vi "加标回收启动 (子VI).vi"(11 "启动参数":T1(ring)=enum."CODCr") -> (0 "error out":T2={"status"=FALSE, "代码"=4, "source"=""} caption="错误输出" {"代码" items=["执行成功"=1, "执行失败，但不知道原因"=2, "命令请求条件错误"=3, "通讯超时"=4, "系统繁忙不能执行"=5, "系统故障"=6, "没有数据"=100]})   [LabVIEW 2016]
uses:
  PLC/PLC.lvlib
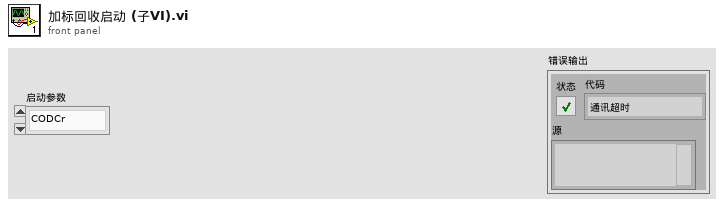
[diagram p1: front panel]
types:
  T1 = enum16{"未选择", "CODMn", "氨氮", "总磷", "总氮", "CODCr"}
  T2 = cluster{"status":bool, "代码":u16, "source":string}
  T3 = enum16{"空闲", "水样测试", "标样核查", "零点核查", "跨度核查", "空白测试", "平行样测试", "质控样", "空白校准", "标样校准", "加标回收"}
  T4 = enum16{"空闲", "水样测试", "标样核查", "零点核查", "跨度核查", "空白测试", "平行样测试", "加标回收", "空白校准", "标样校准", "初始化（清洗）"}
  T5 = cluster{"是否启用仪器":bool, "CODMn":cluster{"启动测量模式":cluster{"测量模式":enum16{"水样测量", "标样核查", "加标回收", "平行样", "校零", "校标"}}, "确定按钮":bool}, "启动模块":cluster{"氨氮":bool, "总磷":bool, "总氮":bool, "COD":bool}, "常规启动":bool, "直接启动":bool}
  T6 = cluster{"R0":i16, "R1":i16, "R2":i16, "R3":i16, "R4":i16, "R5":i16, "R6":i16, "R7":i16, "R8":i16, "R9":i16, "R10":i16, "R11":i16, "R12":i16, "R13":i16, "R14":i16, "R15":i16, "R16":i16, "R17":i16, "R18":i16, "R19":i16, "R20":i16, "R21":i16, "R22":i16, "R23":i16, "R24":i16, "R25":i16, "R26":i16, "R27":i16, "R28":i16, "R29":i16, "R30":i16, "R31":i16, "R32":i16, "R33":i16, "R34":i16, "R35":i16, "R36":i16, "R37":i16, "R38":i16, "R39":i16, "R40":i16, "R41":i16, "R42":i16, "R43":i16, "R44":i16, "R45":i16, "R46":i16, "R47":i16, "R48":i16, "R49":i16, "R50":i16, "R51":i16, "R52":i16, "R53":i16, "R54":i16, "R55":i16, "R56":i16}
  T7 = enum32{"Bad", "Idle", "Run top level", "Running"}
  T8 = cluster{"系统时间":timestamp, "工作状态":enum16{"空闲", "水样测试", "标样核查", "零点核查", "跨度核查", "空白测试", "平行样测试", "加标回收", "空白校准", "标样校准", "初始化（清洗）"}, "测量模式":enum16{"待机", "连续模式", "周期模式", "定点模式", "受控模式", "手动模式"}, "告警代码":u16, "故障代码":u16, "日志代码":u16, "软件版本":u16, "F0":sgl, "F1":sgl, "F2":sgl, "F3":sgl, "T":sgl, "H":sgl, "id":u16, "flowid":u16, "量程":u16, "总磷控温温度1":sgl, "营养盐控温温度2":sgl, "ADC":sgl}
  T9 = cluster{"系统时间":timestamp, "工作状态":u16, "测量模式":u16, "告警代码":enum16{"无告警", "缺试剂告警", "缺水样告警", "缺蒸馏水告警", "缺标液告警", "仪表漏液告警", "标定异常告警", "超量程告警", "加热异常", "低试剂预警", "超上限告警", "超下限告警", "仪表内部其他异常", "滴定异常告警", "电极异常告警", "量程切换告警", "参数设置告警", "PH电极电位异常", "电导率电极异常", "浊度光度异常", "溶解氧电极异常", "溶解氧光强异常", "温度异常告警", "PH异常告警", "溶解氧异常告警", "电导率异常告警", "浊度异常告警", "叶绿素异常告警", "藻密度异常告警", "蓝绿藻异常告警", "ORP异常告警", "氨氮异常告警", "清洁刷异常告警", "SD卡异常告警", "蓝牙异常告警", "Wifi异常告警", "流程异常告警"}, "故障代码":enum16{"无故障", "电机故障", "温度故障", "通讯故障", "滴定故障"}, "日志代码":u16, "软件版本":u16, "F0":sgl, "F1":sgl, "F2":sgl, "F3":sgl, "T":sgl, "H":sgl, "id":u16, "flowid":u16, "量程":u16}
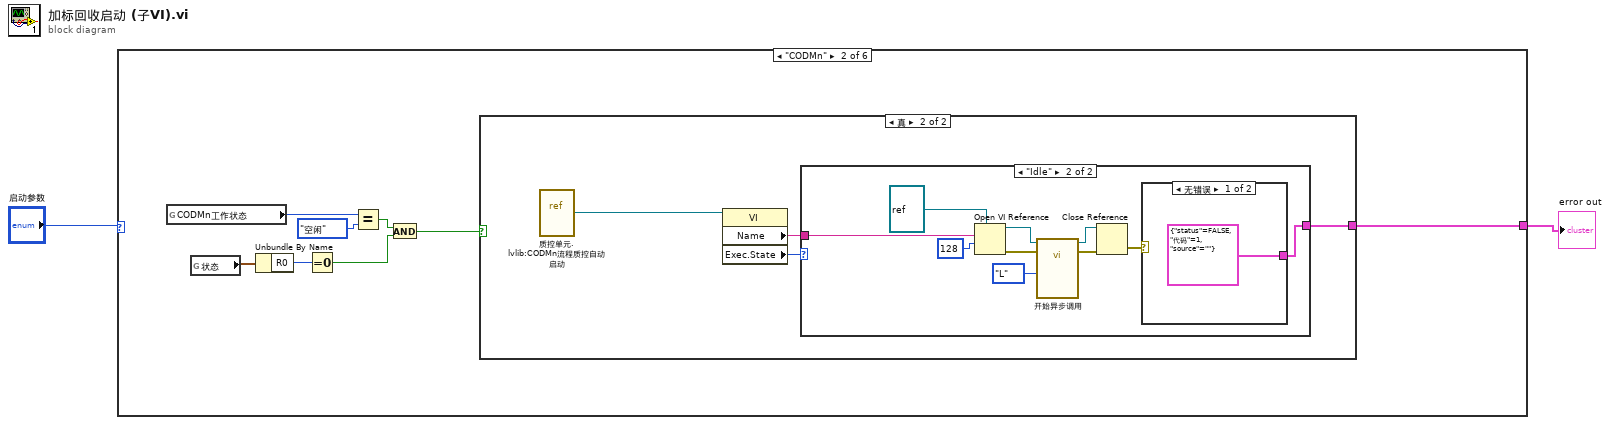
[diagram p0: block diagram]
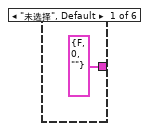
[diagram p2: hidden frame]
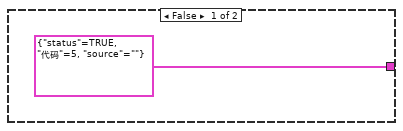
[diagram p3: hidden frame]
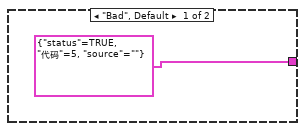
[diagram p4: hidden frame]
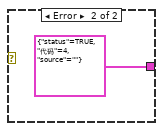
[diagram p5: hidden frame]
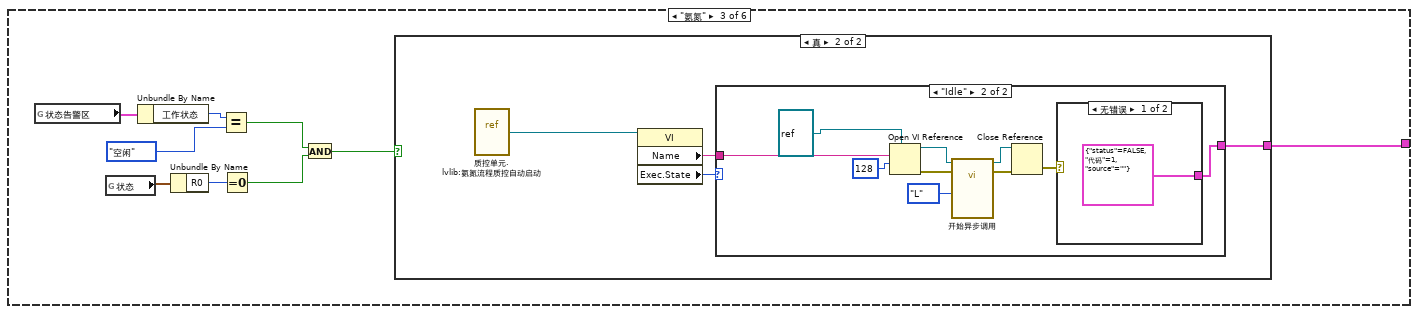
[diagram p6: hidden frame]
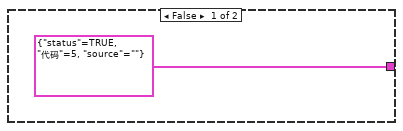
[diagram p7: hidden frame]
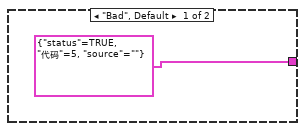
[diagram p8: hidden frame]
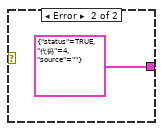
[diagram p9: hidden frame]
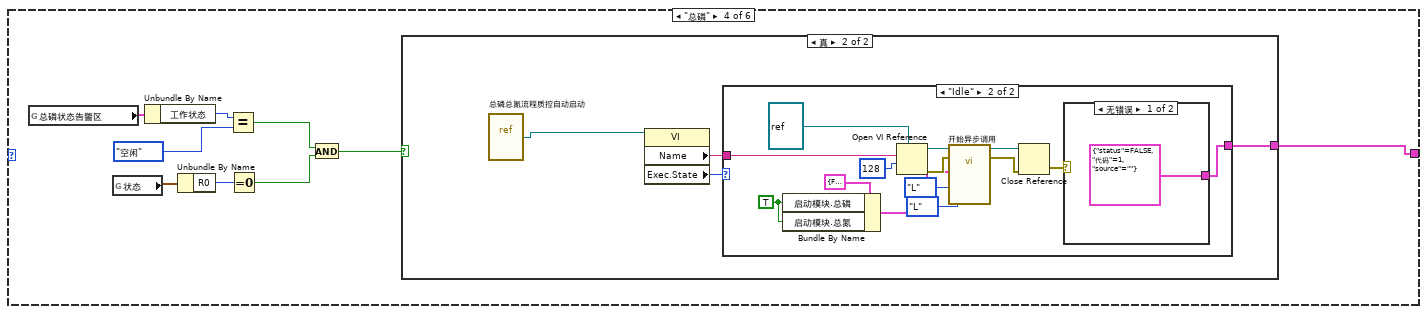
[diagram p10: hidden frame]
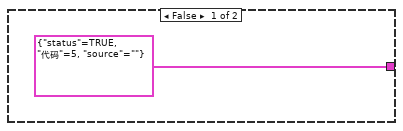
[diagram p11: hidden frame]
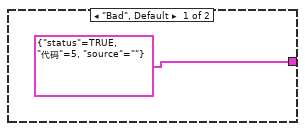
[diagram p12: hidden frame]
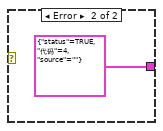
[diagram p13: hidden frame]
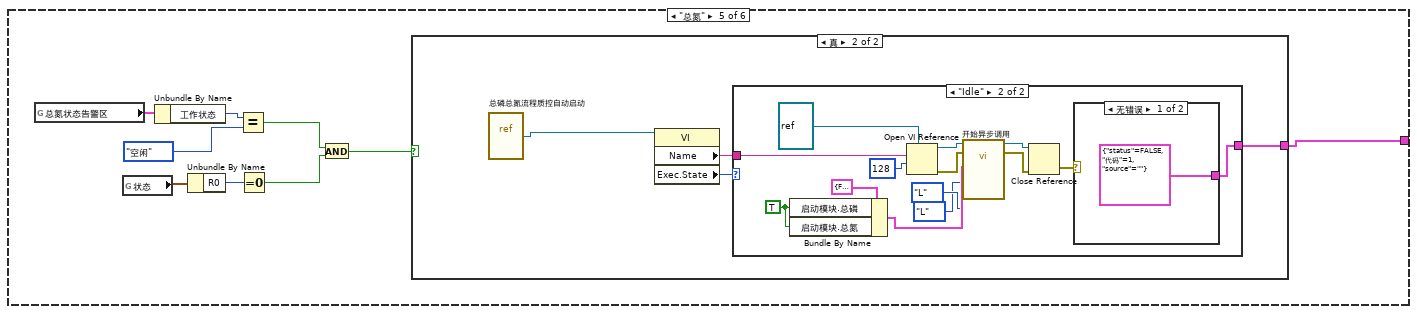
[diagram p14: hidden frame]
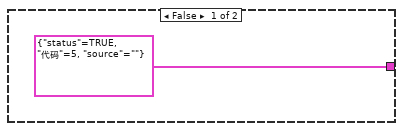
[diagram p15: hidden frame]
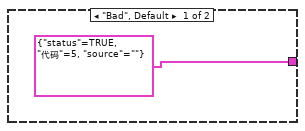
[diagram p16: hidden frame]
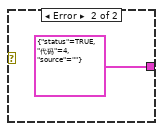
[diagram p17: hidden frame]
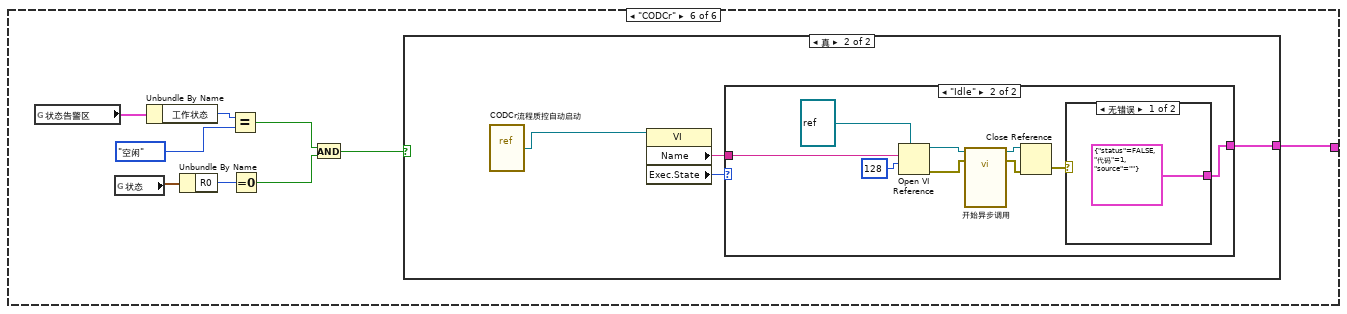
[diagram p18: hidden frame]
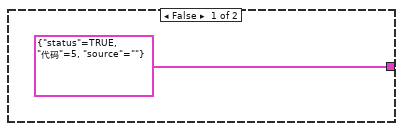
[diagram p19: hidden frame]
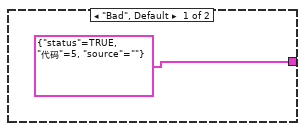
[diagram p20: hidden frame]
diagram:
  n1 = case shown="\"CODMn\"" "启动参数" {
    tunnel: [T2 {"status"=FALSE, "代码"=0, "source"=""} ("error out") w4 w34 w58 w88 w120] -> w1
    frame "未选择", Default {
    }
    frame "CODMn" {
      n2 = global read "COD测量模式全局.vi" "CODMn工作状态"() -> (w11:T3)
      n3 = global read "采配水全局变量.vi" "状态"() -> (w8:T6)
      n4 = Unbundle By Name(w8) -> ("R0"=w7:i16)
      n5 = Equal To 0?(x=w7) -> (x = 0?=w6:bool)
      n6 = Equal?(x=w11, y=T3."空闲") -> (x = y?=w9:bool)
      n7 = And(x=w9, y=w6) -> (x .and. y?=w5:bool)
      n8 = case shown="真" w5 {
        tunnel: [T2 {"status"=TRUE, "代码"=5, "source"=""} ("error out") w13] -> w4
        frame False {
        }
        frame True {
          n9 = vi-ref "质控单元.lvlib:CODMn流程质控自动启动.vi"() -> (w14:refnum<vi>)
          n10 = property class="VI"(reference=w14) -> ("Name"=w16:string, "Exec.State"=w15:T7)  [unwired: 1 in, 2 out]
          n11 = case shown="\"Idle\"" w15 {
            tunnel: w16 -> [_ w24]
            tunnel: [T2 {"status"=TRUE, "代码"=5, "source"=""} ("error out") w20] -> w13
            frame "Bad", Default {
            }
            frame "Idle" {
              n12 = Open VI Reference(type specifier VI Refnum (for type only)=refnum<vi> refnum ("类型说明符VI引用句柄（仅用于类型）"), vi path=w24, options=128 ("选项")) -> (vi reference=w19:refnum<vi>, error out=w23:errorcluster)  [unwired: 3 in]
              n13 = call-by-ref "开始异步调用"(reference=w19, error in=w23, "CODMn量程切换"=enum32{"H", "L", "AUTO"}."L") -> (reference out=w27:refnum<vi>, error out=w22:errorcluster)  [unwired: 10 in]
              n14 = Close Reference(reference=w27, error in (no error)=w22) -> (error out=w21:errorcluster)
              n15 = case shown="无错误" w21 {
                tunnel: [T2 {"status"=FALSE, "代码"=1, "source"=""} ("error out") T2 {"status"=TRUE, "代码"=4, "source"=""} ("error out")] -> w20
                frame No Error {
                }
                frame Error {
                }
              }
            }
          }
        }
      }
    }
    frame "氨氮" {
      n16 = global read "VAR氨氮全局变量.vi" "状态告警区"() -> (w33:T8)
      n17 = global read "采配水全局变量.vi" "状态"() -> (w38:T6)
      n18 = Unbundle By Name(w33) -> ("工作状态"=w32:T4)
      n19 = Unbundle By Name(w38) -> ("R0"=w37:i16)
      n20 = Equal?(x=w32, y=T4."空闲") -> (x = y?=w30:bool)
      n21 = Equal To 0?(x=w37) -> (x = 0?=w36:bool)
      n22 = And(x=w30, y=w36) -> (x .and. y?=w35:bool)
      n23 = case shown="真" w35 {
        tunnel: [T2 {"status"=TRUE, "代码"=5, "source"=""} ("error out") w41] -> w34
        frame False {
        }
        frame True {
          n24 = vi-ref "质控单元.lvlib:氨氮流程质控自动启动.vi"() -> (w40:refnum<vi>)
          n25 = property class="VI"(reference=w40) -> ("Name"=w43:string, "Exec.State"=w42:T7)  [unwired: 1 in, 2 out]
          n26 = case shown="\"Idle\"" w42 {
            tunnel: w43 -> [_ w51]
            tunnel: [T2 {"status"=TRUE, "代码"=5, "source"=""} ("error out") w47] -> w41
            frame "Bad", Default {
            }
            frame "Idle" {
              n27 = Open VI Reference(type specifier VI Refnum (for type only)=refnum<vi> refnum ("类型说明符VI引用句柄（仅用于类型）"), vi path=w51, options=128 ("选项")) -> (vi reference=w54:refnum<vi>, error out=w50:errorcluster)  [unwired: 3 in]
              n28 = call-by-ref "开始异步调用"(reference=w54, error in=w50, "氨氮量程切换"=enum32{"H", "L", "AUTO"}."L") -> (reference out=w53:refnum<vi>, error out=w49:errorcluster)  [unwired: 11 in]
              n29 = Close Reference(reference=w53, error in (no error)=w49) -> (error out=w48:errorcluster)
              n30 = case shown="无错误" w48 {
                tunnel: [T2 {"status"=FALSE, "代码"=1, "source"=""} ("error out") T2 {"status"=TRUE, "代码"=4, "source"=""} ("error out")] -> w47
                frame No Error {
                }
                frame Error {
                }
              }
            }
          }
        }
      }
    }
    frame "总磷" {
      n31 = global read "VAR总磷总氮全局变量.vi" "总磷状态告警区"() -> (w57:T8)
      n32 = global read "采配水全局变量.vi" "状态"() -> (w65:T6)
      n33 = Unbundle By Name(w57) -> ("工作状态"=w61:T4)
      n34 = Unbundle By Name(w65) -> ("R0"=w64:i16)
      n35 = Equal?(x=w61, y=T4."空闲") -> (x = y?=w59:bool)
      n36 = Equal To 0?(x=w64) -> (x = 0?=w63:bool)
      n37 = And(x=w59, y=w63) -> (x .and. y?=w62:bool)
      n38 = case shown="真" w62 {
        tunnel: [T2 {"status"=TRUE, "代码"=5, "source"=""} ("error out") w68] -> w58
        frame False {
        }
        frame True {
          n39 = vi-ref "总磷总氮流程质控自动启动.vi"() -> (w67:refnum<vi>)
          n40 = property class="VI"(reference=w67) -> ("Name"=w70:string, "Exec.State"=w69:T7)  [unwired: 1 in, 2 out]
          n41 = case shown="\"Idle\"" w69 {
            tunnel: w70 -> [_ w84]
            tunnel: [T2 {"status"=TRUE, "代码"=5, "source"=""} ("error out") w81] -> w68
            frame "Bad", Default {
            }
            frame "Idle" {
              w75 = TRUE ("启动模块.总磷")
              n42 = Bundle By Name(cluster=T5 {"是否启用仪器"=FALSE, "CODMn"={"启动测量模式"={"测量模式"=enum."水样测量"}, "确定按钮"=FALSE}, "启动模块"={"氨氮"=FALSE, "总磷"=FALSE, "总氮"=FALSE, "COD"=FALSE}, "常规启动"=FALSE, "直接启动"=FALSE} ("参数"), "启动模块.总磷"=w75, "启动模块.总氮"=w75) -> (w74:T5)
              n43 = Open VI Reference(type specifier VI Refnum (for type only)=refnum<vi> refnum ("类型说明符VI引用句柄（仅用于类型）"), vi path=w84, options=128 ("选项")) -> (vi reference=w79:refnum<vi>, error out=w78:errorcluster)  [unwired: 3 in]
              n44 = call-by-ref "开始异步调用"(reference=w79, error in=w78, "总磷量程切换"=enum32{"H", "L", "AUTO"}."L", "总氮量程切换"=enum32{"H", "L", "AUTO"}."L", "参数"=w74) -> (reference out=w77:refnum<vi>, error out=w83:errorcluster)  [unwired: 9 in]
              n45 = Close Reference(reference=w77, error in (no error)=w83) -> (error out=w82:errorcluster)
              n46 = case shown="无错误" w82 {
                tunnel: [T2 {"status"=FALSE, "代码"=1, "source"=""} ("error out") T2 {"status"=TRUE, "代码"=4, "source"=""} ("error out")] -> w81
                frame No Error {
                }
                frame Error {
                }
              }
            }
          }
        }
      }
    }
    frame "总氮" {
      n47 = global read "VAR总磷总氮全局变量.vi" "总氮状态告警区"() -> (w89:T8)
      n48 = global read "采配水全局变量.vi" "状态"() -> (w96:T6)
      n49 = Unbundle By Name(w89) -> ("工作状态"=w92:T4)
      n50 = Unbundle By Name(w96) -> ("R0"=w95:i16)
      n51 = Equal?(x=w92, y=T4."空闲") -> (x = y?=w90:bool)
      n52 = Equal To 0?(x=w95) -> (x = 0?=w94:bool)
      n53 = And(x=w90, y=w94) -> (x .and. y?=w93:bool)
      n54 = case shown="真" w93 {
        tunnel: [T2 {"status"=TRUE, "代码"=5, "source"=""} ("error out") w99] -> w88
        frame False {
        }
        frame True {
          n55 = vi-ref "总磷总氮流程质控自动启动.vi"() -> (w98:refnum<vi>)
          n56 = property class="VI"(reference=w98) -> ("Name"=w101:string, "Exec.State"=w100:T7)  [unwired: 1 in, 2 out]
          n57 = case shown="\"Idle\"" w100 {
            tunnel: w101 -> [_ w115]
            tunnel: [T2 {"status"=TRUE, "代码"=5, "source"=""} ("error out") w113] -> w99
            frame "Bad", Default {
            }
            frame "Idle" {
              w106 = TRUE ("启动模块.总磷")
              n58 = Bundle By Name(cluster=T5 {"是否启用仪器"=FALSE, "CODMn"={"启动测量模式"={"测量模式"=enum."水样测量"}, "确定按钮"=FALSE}, "启动模块"={"氨氮"=FALSE, "总磷"=FALSE, "总氮"=FALSE, "COD"=FALSE}, "常规启动"=FALSE, "直接启动"=FALSE} ("参数"), "启动模块.总磷"=w106, "启动模块.总氮"=w106) -> (w105:T5)
              n59 = Open VI Reference(type specifier VI Refnum (for type only)=refnum<vi> refnum ("类型说明符VI引用句柄（仅用于类型）"), vi path=w115, options=128 ("选项")) -> (vi reference=w111:refnum<vi>, error out=w110:errorcluster)  [unwired: 3 in]
              n60 = call-by-ref "开始异步调用"(reference=w111, error in=w110, "总磷量程切换"=enum32{"H", "L", "AUTO"}."L" ("总氮量程切换"), "总氮量程切换"=enum32{"H", "L", "AUTO"}."L" ("总磷量程切换"), "参数"=w105) -> (reference out=w109:refnum<vi>, error out=w108:errorcluster)  [unwired: 9 in]
              n61 = Close Reference(reference=w109, error in (no error)=w108) -> (error out=w114:errorcluster)
              n62 = case shown="无错误" w114 {
                tunnel: [T2 {"status"=FALSE, "代码"=1, "source"=""} ("error out") T2 {"status"=TRUE, "代码"=4, "source"=""} ("error out")] -> w113
                frame No Error {
                }
                frame Error {
                }
              }
            }
          }
        }
      }
    }
    frame "CODCr" {
      n63 = global read "CODcr全局变量.vi" "状态告警区"() -> (w119:T9)
      n64 = global read "采配水全局变量.vi" "状态"() -> (w127:T6)
      n65 = Unbundle By Name(w119) -> ("工作状态"=w123:u16)
      n66 = Unbundle By Name(w127) -> ("R0"=w126:i16)
      n67 = Equal?(x=w123, y=T4."空闲") -> (x = y?=w121:bool)
      n68 = Equal To 0?(x=w126) -> (x = 0?=w125:bool)
      n69 = And(x=w121, y=w125) -> (x .and. y?=w124:bool)
      n70 = case shown="真" w124 {
        tunnel: [T2 {"status"=TRUE, "代码"=5, "source"=""} ("error out") w130] -> w120
        frame False {
        }
        frame True {
          n71 = vi-ref "CODCr流程质控自动启动.vi"() -> (w129:refnum<vi>)
          n72 = property class="VI"(reference=w129) -> ("Name"=w132:string, "Exec.State"=w131:T7)  [unwired: 1 in, 2 out]
          n73 = case shown="\"Idle\"" w131 {
            tunnel: w132 -> [_ w141]
            tunnel: [T2 {"status"=TRUE, "代码"=5, "source"=""} ("error out") w139] -> w130
            frame "Bad", Default {
            }
            frame "Idle" {
              n74 = Open VI Reference(type specifier VI Refnum (for type only)=refnum<vi> refnum ("类型说明符VI引用句柄（仅用于类型）"), vi path=w141, options=128 ("选项")) -> (vi reference=w137:refnum<vi>, error out=w136:errorcluster)  [unwired: 3 in]
              n75 = call-by-ref "开始异步调用"(reference=w137, error in=w136) -> (reference out=w135:refnum<vi>, error out=w134:errorcluster)  [unwired: 11 in]
              n76 = Close Reference(reference=w135, error in (no error)=w134) -> (error out=w140:errorcluster)
              n77 = case shown="无错误" w140 {
                tunnel: [T2 {"status"=FALSE, "代码"=1, "source"=""} ("error out") T2 {"status"=TRUE, "代码"=4, "source"=""} ("error out")] -> w139
                frame No Error {
                }
                frame Error {
                }
              }
            }
          }
        }
      }
    }
  }
  "error out" <- w1
